vi "Write Byte Stream.vi"(8 "error in (no error)":errorcluster, 10 "Byte Stream":T1, 11 "UTF8 in":refnum<class "UTF-8 String.lvclass">) -> (0 "error out":errorcluster, 3 "UTF8 out":refnum<class "UTF-8 String.lvclass">)   [LabVIEW 2010, in "JKI Unicode.lvlib" / "UTF-8 String.lvclass"]
uses:
  UTF-8 String.lvclass
  Byte Stream.ctl
  UTF-8 String.lvclass/UTF-8 String.ctl
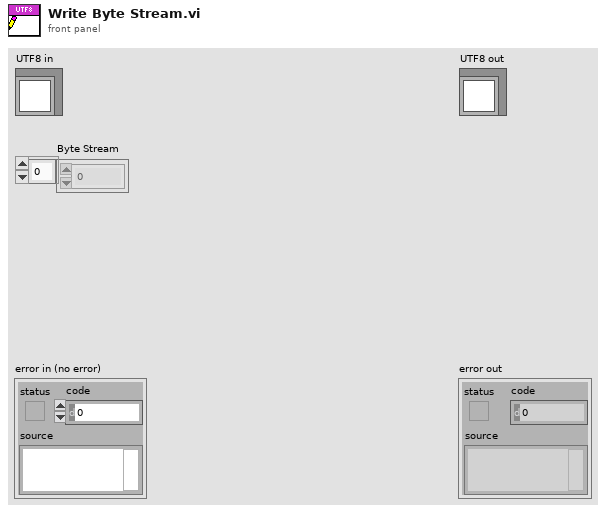
[diagram p1: front panel]
types:
  T1 = typedef "JKI Unicode.lvlib/UTF-8 String.lvclass/Byte Stream.ctl" = u8[]
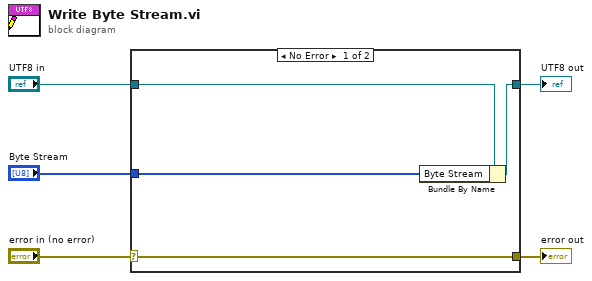
[diagram p0: block diagram]
diagram:
  n1 = case shown="No Error" "error in (no error)" {
    selector: "error in (no error)" -> [w9 w10]
    tunnel: [w9 w10] -> w4
    tunnel: [w7 w11] -> w2
    tunnel: "UTF8 in" -> [w8 w11]
    tunnel: "Byte Stream" -> [w6 _]
    frame No Error {
      n2 = Bundle By Name(cluster=w8, "Byte Stream"=w6) -> (w7:refnum<class "UTF-8 String.lvclass">)
    }
    frame Error {
    }
  }
  "error out" <- w4
  "UTF8 out" <- w2
